vi "StringQueueStateMachine with Error Handler.vi"(8 "ErrI":errorcluster) -> (0 "ErrO":errorcluster)   [LabVIEW 2020]
panel:
  in  "OK":bool
  in  "Exit":bool
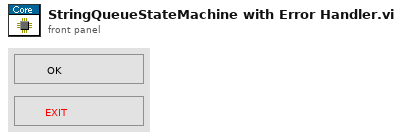
[diagram p1: front panel]
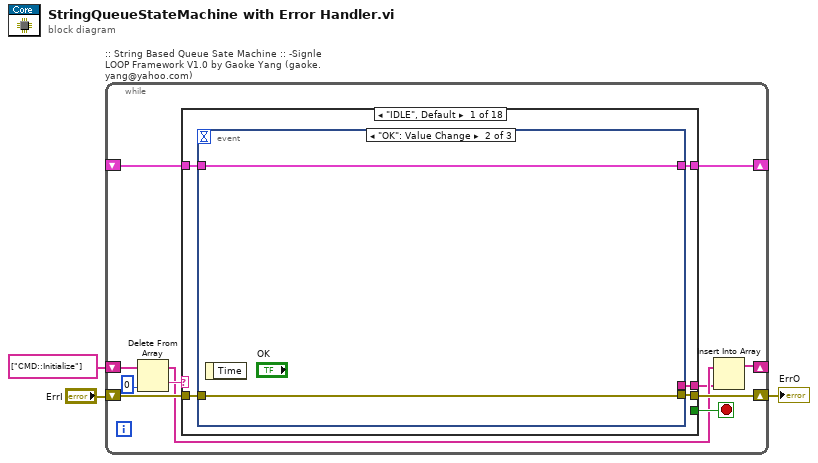
[diagram p0: block diagram]
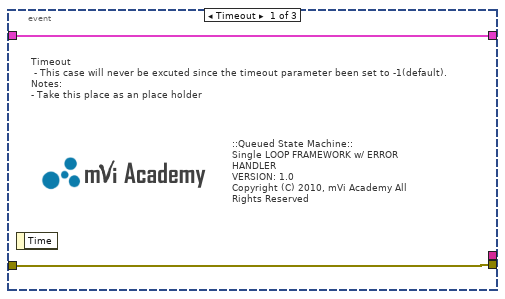
[diagram p2: hidden frame]
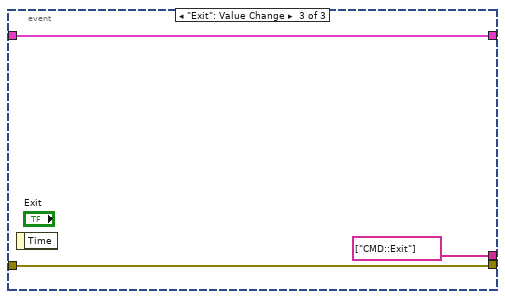
[diagram p3: hidden frame]
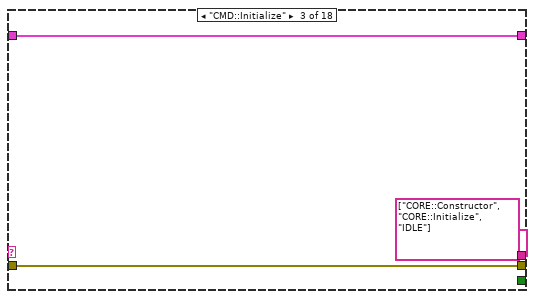
[diagram p5: hidden frame]
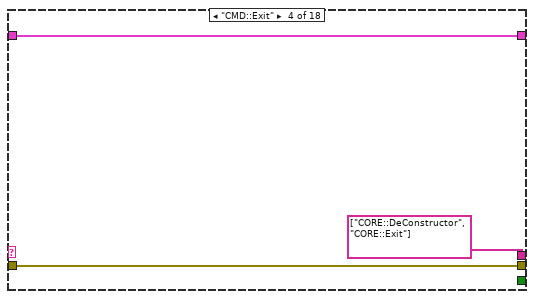
[diagram p6: hidden frame]
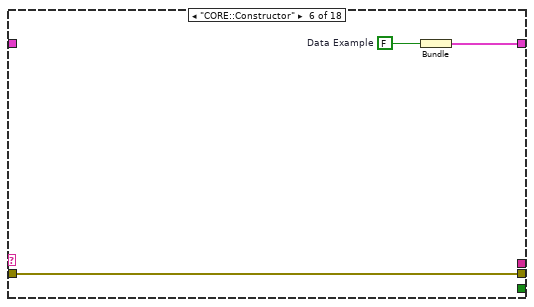
[diagram p8: hidden frame]
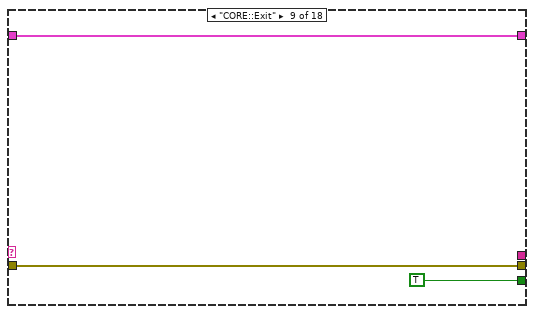
[diagram p11: hidden frame]
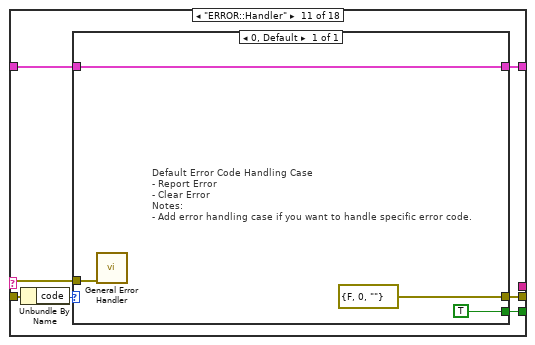
[diagram p13: hidden frame]
diagram:
  n1 = while ":: String Based Queue Sate Machine :: -Signle LOOP Framework V1.0 by Gaoke Yang (gaoke.yang@yahoo.com)" {
    shift-right: [w11] -> w3
    shift-left: "ErrI" -> [w9]
    shift-right: [w13] -> _
    shift-left: _ -> [w12]
    shift-right: [w4] -> _
    shift-left: string[] ["CMD::Initialize"] -> [w10]
    stop <- w14 stop-if-true
    n2 = Delete From Array(array=w10, index=0) -> (deleted portion=w8:string, array with subset deleted=w6:string[])  [unwired: 1 in]
    n3 = case shown="\"IDLE\", Default" w8 {
      tunnel: [w18 w28 w30 w33 w36 w39 w41 w43 w44 w48 w51 w59 w61 w63 w66 w68 w70 w71] -> w11
      tunnel: [_ _ _ _ _ _ _ _ TRUE _ w50 _ _ _ _ _ _ _] -> w14
      tunnel: w9 -> [w19 w28 w30 w33 w36 w39 w41 w43 w44 w48 w49 w59 w61 w63 w66 w68 w70 w71]
      tunnel: [w16 w27 w31 w34 w35 w37 w40 w42 w45 w47 w52 w60 w62 w64 w65 w67 w69 w72] -> w13
      tunnel: w12 -> [w17 w27 w31 w34 w35 _ w40 w42 w45 w47 w53 w60 w62 w64 w65 w67 w69 w72]
      tunnel: [w15 _ string[] ["CORE::Constructor", "CORE::Initialize", "IDLE"] string[] ["CORE::DeConstructor", "CORE::Exit"] _ _ _ _ _ _ _ _ _ _ _ _ _ _] -> w5
      frame "IDLE", Default {
        n4 = event shown="[1] \"OK\": Value Change" {
          selector: _ -> [_ _ _]
          dyn-events: _ -> [_ _ _]
          timeout: _ -> [_ _ _]
          tunnel: [w21 w23 w26] -> w18
          tunnel: w19 -> [w21 w23 w26]
          tunnel: [w20 w22 w25] -> w16
          tunnel: w17 -> [w20 w22 w25]
          tunnel: [_ _ string[] ["CMD::Exit"]] -> w15
          event Timeout {
            # "Timeout\n - This case will never be excuted since the timeout parameter been set to -1(default).\nNotes:\n- Take this place as an place holder"
            # "::Queued State Machine::\nSingle LOOP FRAMEWORK w/ ERROR HANDLER\nVERSION: 1.0\nCopyright (C) 2010, mVi Academy All Rights Reserved"
            n5 = event-data() -> ()  [unwired: 1 in, 1 out]
          }
          event "OK": Value Change {
            n6 = event-data() -> ()  [unwired: 1 in, 1 out]
          }
          event "Exit": Value Change {
            n7 = event-data() -> ()  [unwired: 1 in, 1 out]
          }
        }
      }
      frame "-------- Commands ---------" {
      }
      frame "CMD::Initialize" {
      }
      frame "CMD::Exit" {
      }
      frame "------------ Core ------------" {
      }
      frame "CORE::Constructor" {
        w38 = FALSE  # Data Example
        n8 = Bundle("Data Example"=w38) -> (w37:cluster{"Data Example":bool})  [unwired: 1 in]
      }
      frame "CORE::Initialize" {
      }
      frame "CORE::DeConstructor" {
      }
      frame "CORE::Exit" {
      }
      frame "-------- Error Handle--------" {
      }
      frame "ERROR::Handler" {
        n9 = Unbundle By Name(w49) -> ("code"=w54:i32)
        n10 = case shown="0, Default" w54 {
          tunnel: [w58] -> w52
          tunnel: w53 -> [w58]
          tunnel: [errorcluster {"status"=FALSE, "code"=0, "source"=""} ("error out")] -> w51
          tunnel: [TRUE] -> w50
          tunnel: w49 -> [w56]
          frame 0, Default {
            # "Default Error Code Handling Case\n- Report Error\n- Clear Error \nNotes:\n- Add error handling case if you want to handle specific error code."
            n11 = call <vilib>:"General Error Handler.vi"("error in (no error)"=w56) -> ()  [unwired: 10 in, 5 out]
          }
        }
      }
      frame "------------  GUI  ------------" {
      }
      frame "GUI::Initialize" {
      }
      frame "GUI::SetCusor" {
      }
      frame "GUI::SetMenu" {
      }
      frame "------------ USER -----------" {
      }
      frame "USER::Case1" {
      }
      frame "USER::Case2" {
      }
    }
    n12 = Insert Into Array(array=w6, new element=w5) -> (w4:string[])  [unwired: 1 in]
  }
  "ErrO" <- w3
